vi "FM_WS_tool.vi"() -> ()   [LabVIEW 2013]
uses:
  <vilib>/NI VeriStand/Execution/Workspace/NI_VS Workspace ExecutionAPI.lvlib
  <vilib>/NI Veristand/Templates/Workspace Tool Support/Workspace Tool Response (String).ctl
  <vilib>/NI VeriStand/Templates/Workspace Tool Support/NI VeriStand - Workspace Tool Support.lvlib
  <vilib>/NI Veristand/Execution/Project/NI_VS Project ExecutionAPI.lvlib
  <vilib>/NI/AMC/AMC.lvlib
  <vilib>/NI Veristand/Execution/Project/Project Ref.ctl
  <vilib>/NI Veristand/Execution/Workspace/NI VeriStand - Get Multiple Channel Values.vi
  <vilib>/NI Veristand/Execution/Project/NI VeriStand - Send Workspace Tool Message (String).vi
  NationalInstruments.VeriStand.ClientAPI
  <vilib>/NI Veristand/Execution/Workspace/WorkspaceAPI.ctl
  NationalInstruments.VeriStand.SystemStorage
  _support/CustomTool_Data.ctl
  <vilib>/NI Veristand/Templates/Workspace Tool Support/Workspace Tool Response (Byte Array).ctl
  <vilib>/NI Veristand/Templates/Workspace Tool Support/Workspace Tool Message (Byte Array).ctl
  <vilib>/NI Veristand/Templates/Workspace Tool Support/Workspace Tool Message (String).ctl
  <vilib>/NI Veristand/Templates/Workspace Tool Support/Workspace Tool Message Bus.ctl
panel:
  out "value sent":dbl
  out "Execution:State (Before)":T1(ring)
  in  "Send Message To Service":bool
  in  "Launch Service":bool
  out "Send Error":errorcluster
  out "SaveSystemStorageFile":bool
  in  "Destination":path
  in  "Save As":bool
  in  "NIVS.Project Doc":refnum<k24>
  in  "Data":string
  out "Command":string
  out "Data":string
  in  "Command":string="Shut Down"
  in  "Custom Tool Path":string="..\\Workspace.vi"
  in  "Send":bool
  out "ShutDown Command?":bool
  in  "NIVS.Message Bus":T2
  in  "NIVS.ProjectRoot":refnum<k24>
  out "Commands Received":i32
  in  "Stop":bool
  in  "NIVS.System Definition Root":refnum<k24>
  in  "NIVS.Project File Path":path
  in  "NIVS.Workspace Event":refnum<event-registration>
  out "System Times":dbl[](array[numeric]) format="%<%H:%M:%S%3u>t"
  in  "NIVS.Gateway IP Address":string
  in  "NIVS.INI File Path":path
  # "Incoming Commands"
  # "Outgoing Commands"
  # "Status"
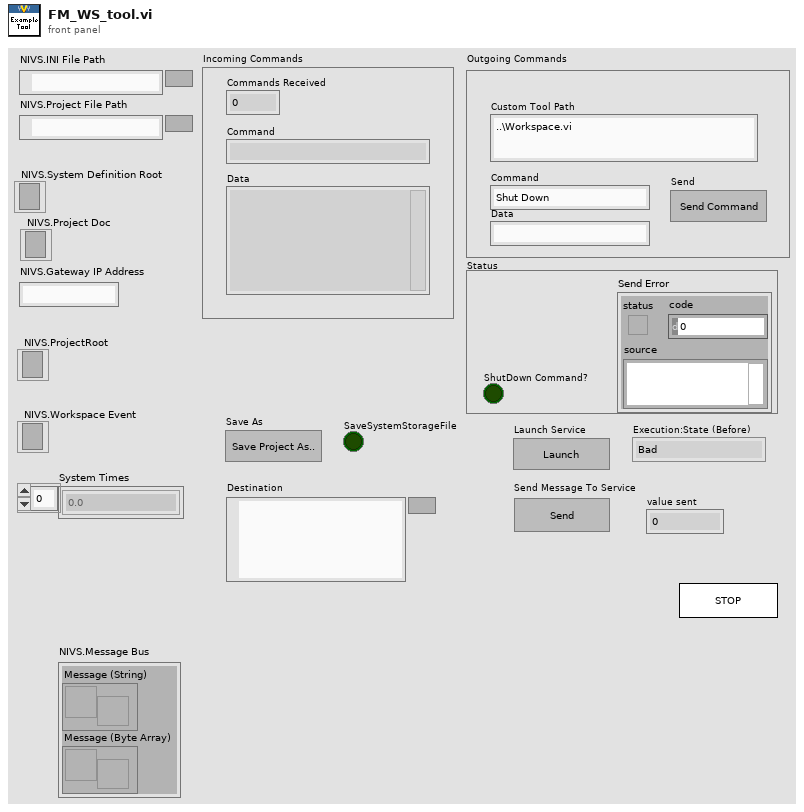
[diagram p1: front panel]
types:
  T1 = enum32{"Bad", "Idle", "Run top level", "Running"}
  T2 = typedef "NI VeriStand - Workspace Tool Support.lvlib/Workspace Tool Message Bus.ctl" = cluster{"Message (String)":refnum<user-event>, "Message (Byte Array)":refnum<user-event>}
  T3 = typedef "CustomTool_Data.ctl" = cluster{"Project Ref":T4, "Log File":path, "WorkspaceManager  out":T5, "NIVS.Project File Path":path, "NIVS.Project Doc":refnum<k24>, "Service Ref":refnum<vi>, "Service Name":string}
  T4 = typedef "NI_VS Project ExecutionAPI.lvlib/Project Ref.ctl" = refnum<k24>
  T5 = typedef "NI_VS Workspace ExecutionAPI.lvlib/WorkspaceAPI.ctl" = refnum<k24>
  T6 = typedef "NI_VS Workspace ExecutionAPI.lvlib/SystemStateEventRef.ctl" = cluster{"CustDatRef":refnum<user-event>, "EvtRef":refnum<k27>}
  T7 = typedef "NI_VS Workspace ExecutionAPI.lvlib/SystemStateRegEventRef.ctl" = refnum<event-registration>
  T8 = typedef "AMC.lvlib/Message Queue.ctl" = refnum<queue>
  T9 = cluster{"NIVS.Workspace Event":refnum<event-registration>, "SystemChangeEventRef":T7, "Event Registration Refnum":refnum<event-registration>}
  T10 = typedef "NI VeriStand - Workspace Tool Support.lvlib/Workspace Tool Response (String).ctl" = cluster{"Response":string, "Error":errorcluster}
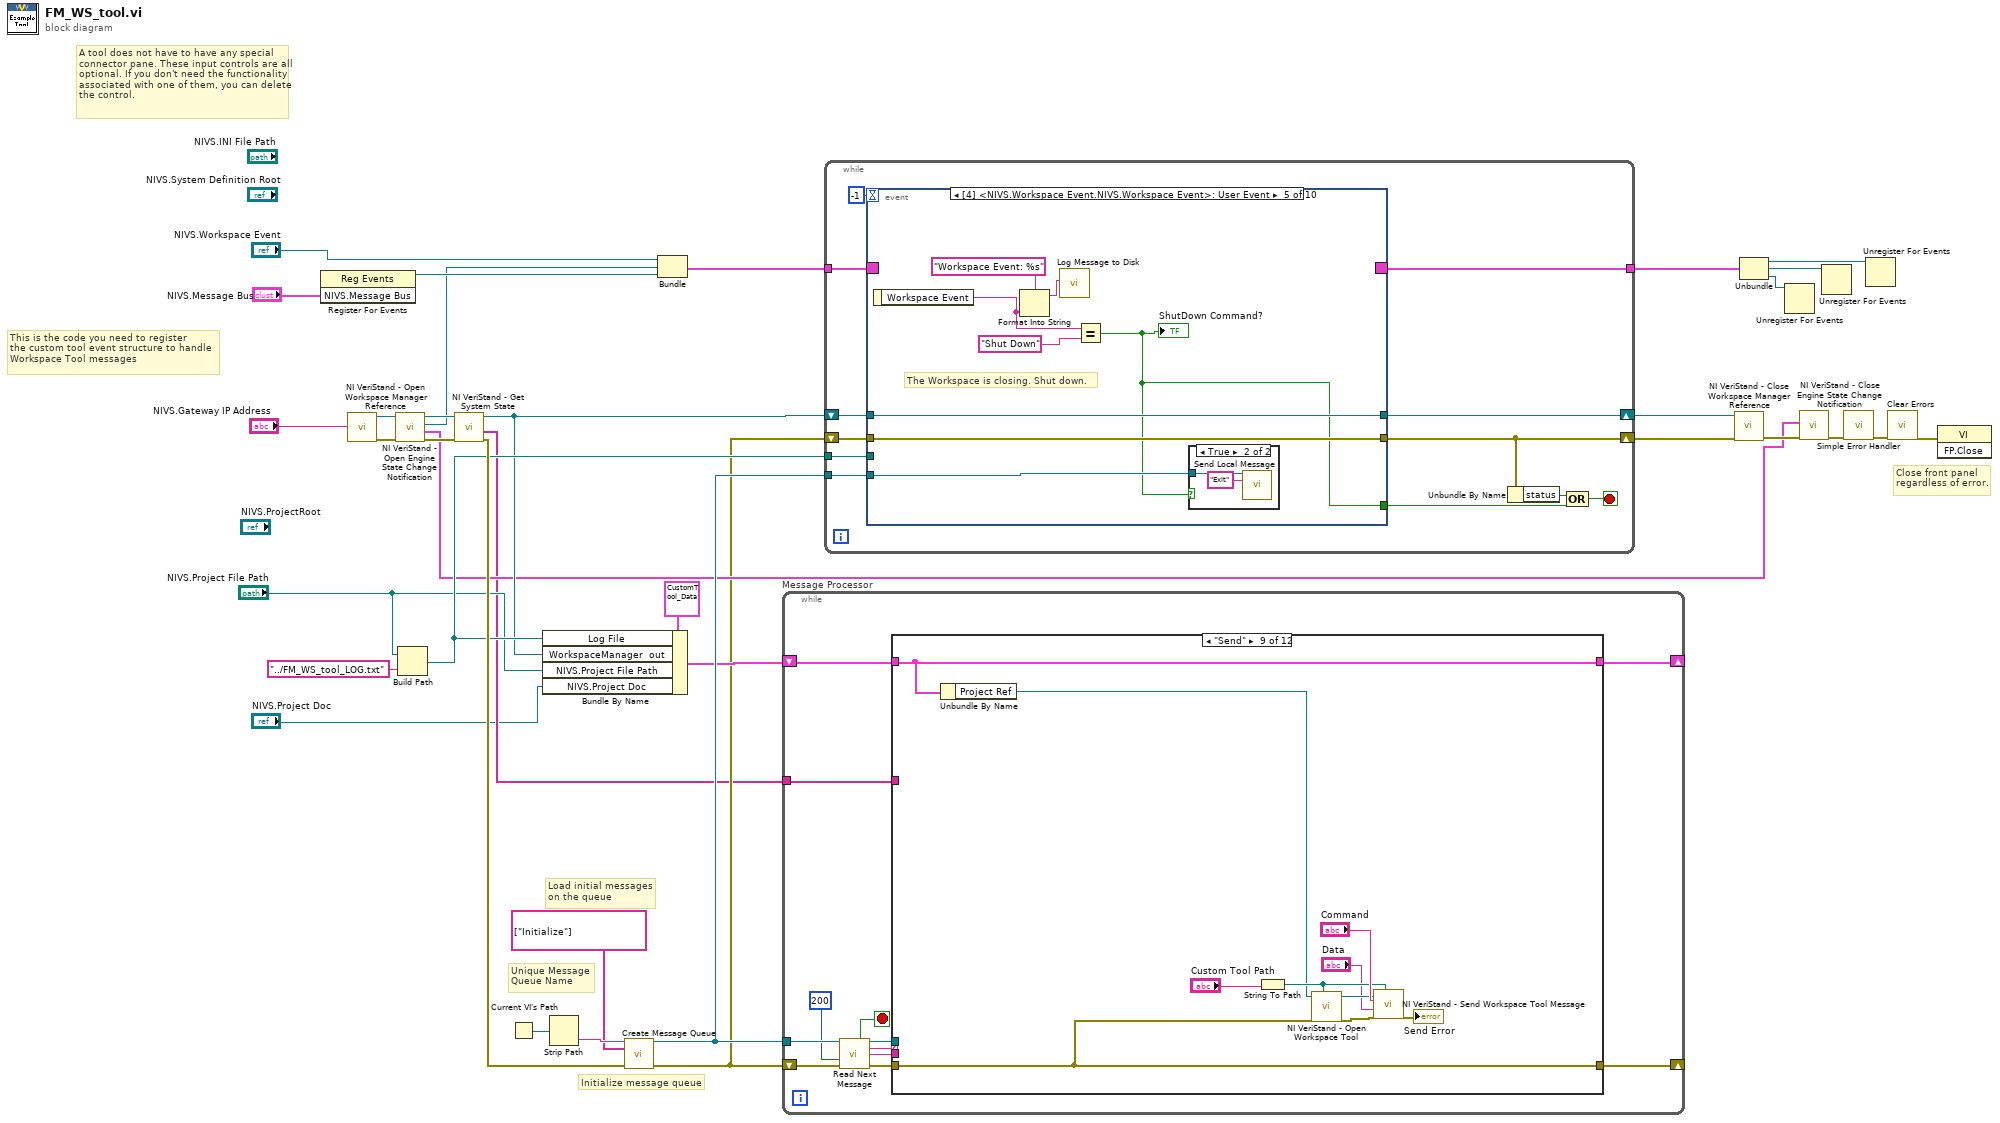
[diagram p0: block diagram]
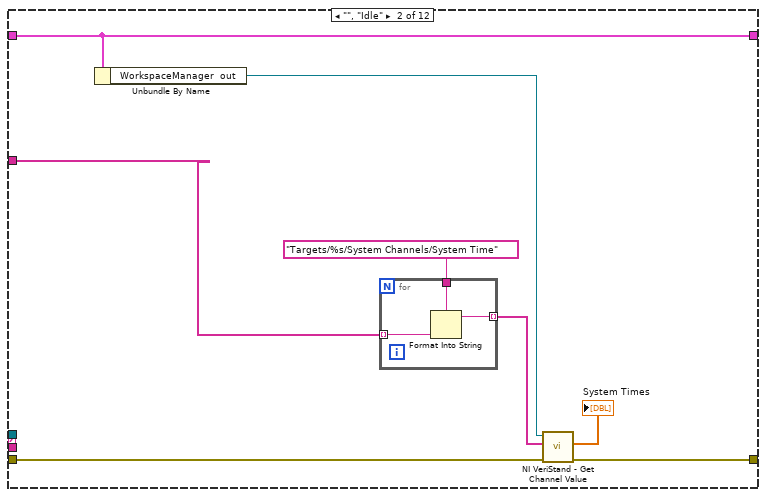
[diagram p3: hidden frame]
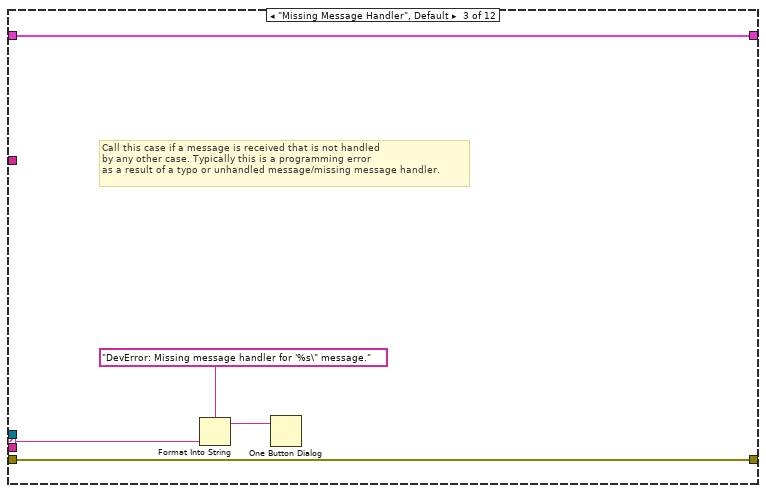
[diagram p4: hidden frame]
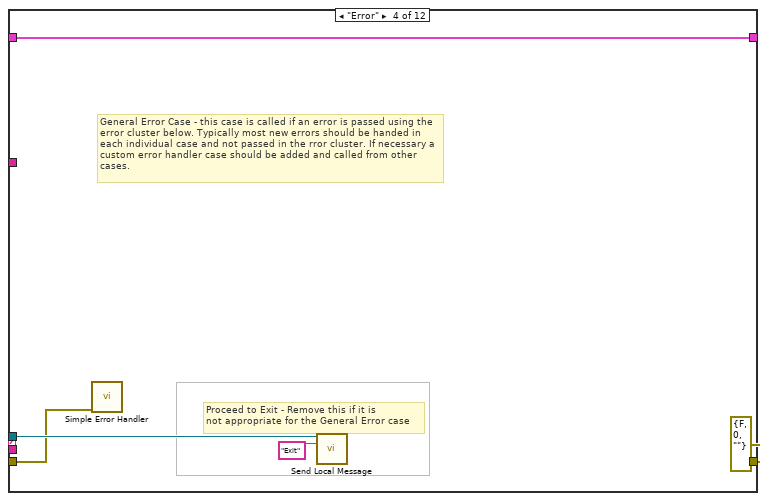
[diagram p5: hidden frame]
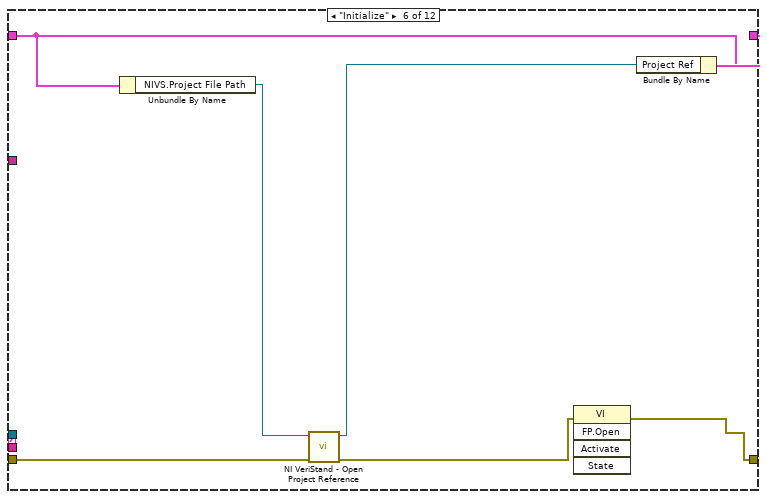
[diagram p7: hidden frame]
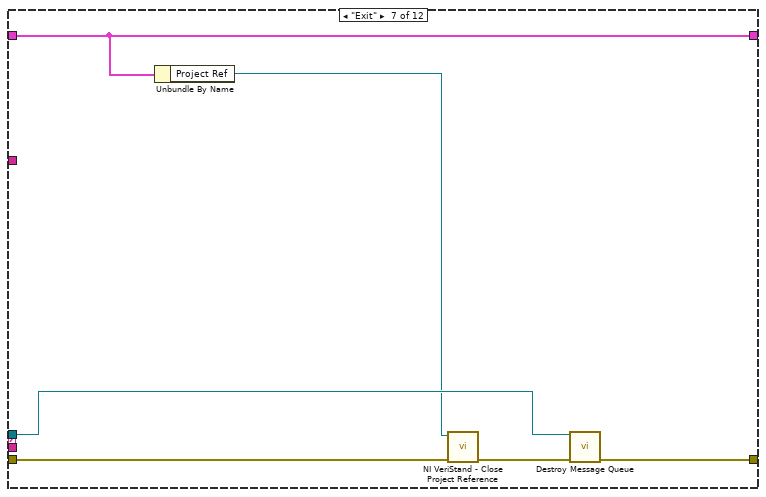
[diagram p8: hidden frame]
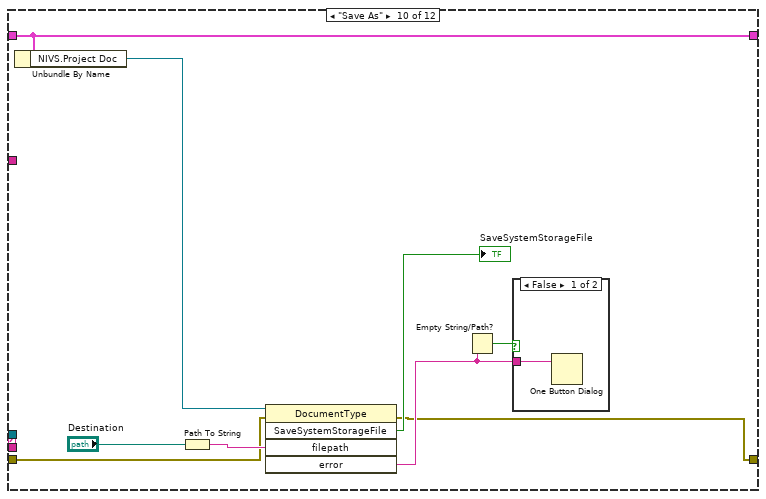
[diagram p10: hidden frame]
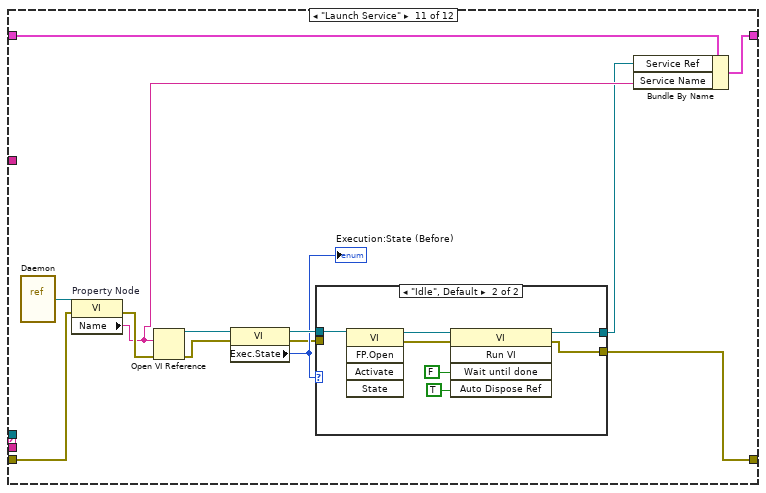
[diagram p12: hidden frame]
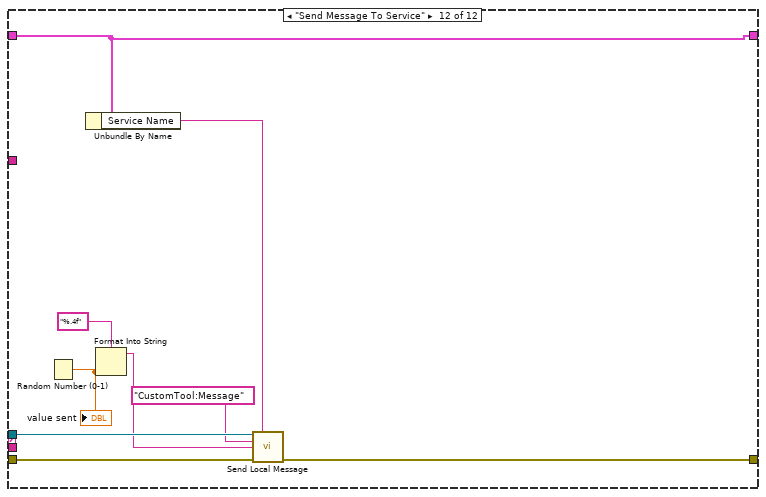
[diagram p14: hidden frame]
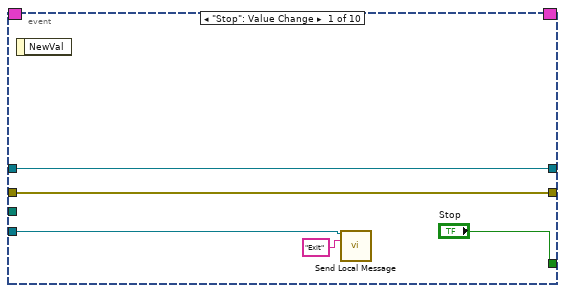
[diagram p15: hidden frame]
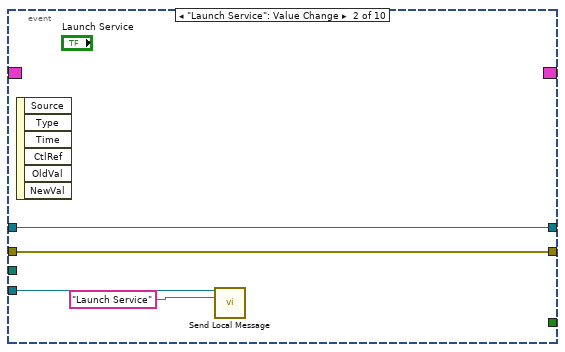
[diagram p16: hidden frame]
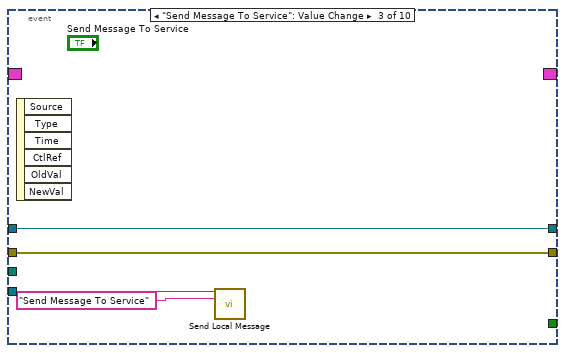
[diagram p17: hidden frame]
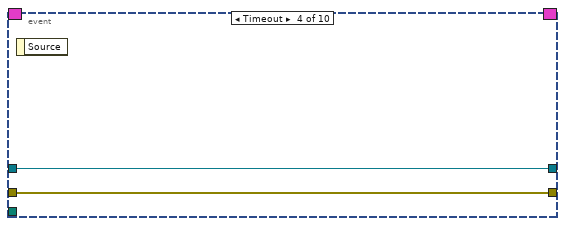
[diagram p18: hidden frame]
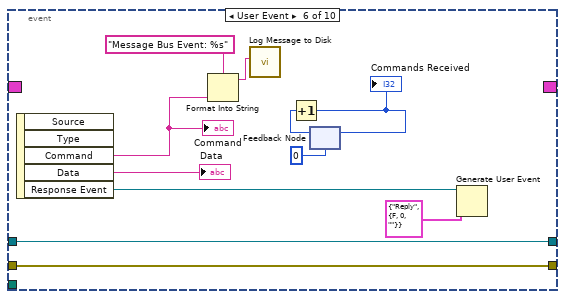
[diagram p20: hidden frame]
diagram:
  # "Initialize message queue"
  # "Unique Message\nQueue Name"
  # "Load initial messages\non the queue"
  # "This is the code you need to register \nthe custom tool event structure to handle\nWorkspace Tool messages"
  # "A tool does not have to have any special connector pane. These input controls are all optional. If you don't need the functionality associated with one of them, you can delete the control."
  # "Close front panel\nregardless of error."
  n1 = register-events("NIVS.Message Bus") -> (reference out=w24:refnum<event-registration>)  [unwired: 2 in, 1 out]
  n2 = call <vilib>:"NI VeriStand - Open Workspace Manager Reference.vi"("Gateway IP Address (\"\": localhost)"="NIVS.Gateway IP Address") -> ("error out"=w15:errorcluster, "WorkspaceManager"=w16:T5)  [unwired: 9 in]
  n3 = call <vilib>:"NI VeriStand - Open Engine State Change Notification.vi"("error in (no error)"=w15, "WorkspaceManager in"=w16) -> ("error out"=w17:errorcluster, "SystemStateRefs"=w5:T6, "SystemChangeEventRef"=w14:T7, "WorkspaceManager out"=w18:T5)  [unwired: 6 in]
  n4 = Build Path(base path="NIVS.Project File Path", name or relative path="../FM_WS_tool_LOG.txt") -> (appended path=w7:path)
  n5 = call <vilib>:"NI VeriStand - Get System State.vi"("error in (no error)"=w17, "WorkspaceManager in"=w18) -> ("error out"=w13:errorcluster, "Targets"=w2:string[], "WorkspaceManager  out"=w6:T5)  [unwired: 5 in, 2 out]
  n6 = Current VI's Path() -> (path=w22:path)
  n7 = Bundle By Name(cluster=T3 {"Project Ref"=refnum, "Log File"=path "", "WorkspaceManager  out"=refnum, "NIVS.Project File Path"=path "", "NIVS.Project Doc"=refnum, "Service Ref"=refnum, "Service Name"=""}, "Log File"=w7, "WorkspaceManager  out"=w6, "NIVS.Project File Path"="NIVS.Project File Path", "NIVS.Project Doc"="NIVS.Project Doc") -> (w8:T3)
  n8 = Strip Path(path=w22) -> (name=w21:string)  [unwired: 1 out]
  n9 = call <vilib>:"Create Message Queue.vi"("message queue name"=w21, "initial message names"=string[] ["Initialize"], "error in"=w13) -> ("message queue out"=w11:T8, "error out"=w4:errorcluster)  [unwired: 11 in]
  n10 = Bundle("NIVS.Workspace Event"="NIVS.Workspace Event", "SystemChangeEventRef"=w14, "Event Registration Refnum"=w24) -> (w33:T9)  [unwired: 1 in]
  n11 = while "Message Processor" {
    shift-left: w4 -> [w41]
    shift-right: [w45] -> _
    tunnel: w11 -> [w42]
    shift-left: w8 -> [w47]
    shift-right: [w46] -> _
    tunnel: w2 -> [w36]
    stop <- w44 stop-if-true
    n12 = call <vilib>:"Read Next Message.vi"("message queue in"=w42, "timeout (1 ms)"=200, "error in"=w41) -> ("exit process?"=w44:bool, "message queue out"=w43:T8, "message name"=w39:string, "message value"=w38:string, "error out"=w40:errorcluster)  [unwired: 5 in, 3 out]
    n13 = case shown="\"Send\"" w39 {
      selector: w39 -> [_ _ w63 _ _ _ _ _ _ _ _ _]
      tunnel: [w49 w57 w65 w70 w72 w78 w83 w87 w89 w99 w108 w131] -> w46
      tunnel: w47 -> [w49 w57 w65 w70 w72 w77 w83 w87 w89 w99 w111 w131]
      tunnel: w43 -> [_ _ _ w68 _ _ w85 _ _ _ _ w138]
      tunnel: w40 -> [w48 w54 w64 w66 w71 w79 w82 w86 w91 w101 w114 w135]
      tunnel: [w48 w53 w64 errorcluster {"status"=FALSE, "code"=0, "source"=""} ("error out") w71 w73 w84 w86 w91 w100 w112 w130] -> w45
      tunnel: w38 -> [_ _ _ _ _ _ _ _ _ _ _ _]
      tunnel: w36 -> [_ w50 _ _ _ _ _ _ _ _ _ _]
      frame "---------- Framework Operations ----------" {
        # "Dummy case to add a seperator in the Case Structure menu"
      }
      frame "", "Idle" {
        n14 = Unbundle By Name(w57) -> ("WorkspaceManager  out"=w51:T5)
        n15 = for {
          tunnel: "Targets/%s/System Channels/System Time" ("format string") -> [w60]
          tunnel: [w59] -> w56 mode=indexing
          tunnel: w50 -> [w58] mode=indexing
          n16 = Format Into String(format string=w60, w58) -> (resulting string=w59:string)  [unwired: 2 in, 1 out]
        }
        n17 = call-poly <vilib>:"NI VeriStand - Get Channel Value.vi"("error in (no error)"=w54, "Channels"=w56, "WorkspaceManager in"=w51) -> ("error out"=w53:errorcluster, "Values"=→"System Times":dbl[])  [unwired: 6 in, 1 out]
      }
      frame "Missing Message Handler", Default {
        # "Call this case if a message is received that is not handled \nby any other case. Typically this is a programming error\nas a result of a typo or unhandled message/missing message handler."
        n18 = Format Into String(format string="DevError: Missing message handler for '%s\" message." ("message"), w63) -> (resulting string=w61:string)  [unwired: 2 in, 1 out]
        n19 = One Button Dialog(message=w61) -> ()  [unwired: 2 out]
      }
      frame "Error" {
        # "Proceed to Exit - Remove this if it is\nnot appropriate for the General Error case"
        # "General Error Case - this case is called if an error is passed using the error cluster below. Typically most new errors should be handed in each individual case and not passed in the rror cluster. If necessary a custom error handler case should be added and called from other cases."
        n20 = call <vilib>:"Simple Error Handler.vi"("error in (no error)"=w66) -> ()  [unwired: 1 in, 8 out]
        n21 = call <vilib>:"Send Local Message.vi"("message queue in"=w68, "message name"="Exit") -> ()  [unwired: 11 in, 3 out]
      }
      frame "---------- Generic Operations ----------" {
        # "Dummy case to add a seperator in the Case Structure menu"
      }
      frame "Initialize" {
        n22 = Unbundle By Name(w77) -> ("NIVS.Project File Path"=w76:path)
        n23 = call <vilib>:"NI VeriStand - Open Project Reference.vi"("error in (no error)"=w79, "Project File Path"=w76) -> ("error out"=w74:errorcluster, "Project Ref"=w75:T4)  [unwired: 8 in]
        n24 = invoke class="VI" method="FP.Open"(error in=w74) -> (error out=w73:errorcluster)  [unwired: 4 in, 4 out]
        n25 = Bundle By Name(cluster=w77, "Project Ref"=w75) -> (w78:T3)
      }
      frame "Exit" {
        n26 = Unbundle By Name(w83) -> ("Project Ref"=w80:T4)
        n27 = call <vilib>:"NI VeriStand - Close Project Reference.vi"("error in (no error)"=w82, "Project Ref"=w80) -> ("error out"=w81:errorcluster)  [unwired: 9 in]
        n28 = call <vilib>:"Destroy Message Queue.vi"("message queue in"=w85, "error in"=w81) -> ("error out"=w84:errorcluster)  [unwired: 11 in, 2 out]
      }
      frame "---------- Application Operations ----------" {
        # "Dummy case to add a seperator in the Case Structure menu"
      }
      frame "Send" {
        n29 = Unbundle By Name(w89) -> ("Project Ref"=w88:T4)
        n30 = String To Path(string="Custom Tool Path") -> (path=w93:path)
        n31 = call <vilib>:"NI VeriStand - Open Workspace Tool.vi"("Workspace Tool Path"=w93, "error in (no error)"=w91, "Project Ref in"=w88) -> ("error out"=w94:errorcluster, "Project Ref out"=w95:T4)  [unwired: 7 in]
        n32 = call-poly <vilib>:"NI VeriStand - Send Workspace Tool Message.vi"("Workspace Tool Path"=w93, "error in (no error)"=w94, "Data"="Data", "Command"="Command", "Project Ref in"=w95) -> ("error out"=→"Send Error":errorcluster)  [unwired: 4 in, 2 out]
      }
      frame "Save As" {
        n33 = Unbundle By Name(w99) -> ("NIVS.Project Doc"=w98:refnum<k24>)
        n34 = Path To String(path="Destination") -> (string=w102:string)
        n35 = invoke class="DocumentType" method="SaveSystemStorageFile"(reference=w98, error in=w101, "filepath"=w102) -> (error out=w100:errorcluster, "SaveSystemStorageFile"=→"SaveSystemStorageFile":bool, "error"=w103:string)  [unwired: 2 in, 2 out]
        n36 = Empty String/Path?(string/path=w103) -> (empty?=w104:bool)
        n37 = case shown="False" w104 {
          tunnel: w103 -> [w107 _]
          frame False {
            n38 = One Button Dialog(message=w107) -> ()  [unwired: 1 in, 1 out]
          }
          frame True {
          }
        }
      }
      frame "Launch Service" {
        n39 = vi-ref "Daemon.vi"() -> (w120:refnum<vi>)
        n40 = property on="Property Node" class="VI"(reference=w120, error in=w114) -> (error out=w113:errorcluster, "Name"=w110:string)  [unwired: 1 out]
        n41 = Open VI Reference(vi path=w110, error in (no error)=w113) -> (vi reference=w119:refnum<vi>, error out=w118:errorcluster)  [unwired: 4 in]
        n42 = property class="VI"(reference=w119, error in=w118) -> (reference out=w117:refnum<vi>, error out=w115:errorcluster, "Exec.State"=w116:T1)
        "Execution:State (Before)" <- w116
        n43 = case shown="\"Idle\", Default" w116 {
          tunnel: w117 -> [w122 w125]
          tunnel: [w122 w124] -> w109
          tunnel: w115 -> [w121 _]
          tunnel: [w121 w123] -> w112
          frame "Run top level" {
          }
          frame "Idle", Default {
            n44 = invoke class="VI" method="FP.Open"(reference=w125) -> (reference out=w127:refnum<vi>, error out=w126:errorcluster)  [unwired: 4 in, 3 out]
            n45 = invoke class="VI" method="Run VI"(reference=w127, error in=w126, "Wait until done"=FALSE ("Auto Dispose Reference"), "Auto Dispose Ref"=TRUE ("Auto Dispose Reference")) -> (reference out=w124:refnum<vi>, error out=w123:errorcluster)  [unwired: 1 in, 3 out]
          }
        }
        n46 = Bundle By Name(cluster=w111, "Service Ref"=w109, "Service Name"=w110) -> (w108:T3)
      }
      frame "Send Message To Service" {
        n47 = Random Number (0-1)() -> (number: 0 to 1=w134:dbl)
        "value sent" <- w134
        n48 = Unbundle By Name(w131) -> ("Service Name"=w137:string)
        n49 = Format Into String(format string="%.4f", w134) -> (resulting string=w132:string)  [unwired: 2 in, 1 out]
        n50 = call <vilib>:"Send Local Message.vi"("message queue in"=w138, "receiver process (\"\" - local)"=w137, "message name"="CustomTool:Message", "message value"=w132, "error in"=w135) -> ("error out"=w130:errorcluster)  [unwired: 8 in, 2 out]
      }
    }
  }
  n51 = while {
    tunnel: w33 -> [w150]
    tunnel: [w149] -> w32
    shift-right: [w144] -> w34
    shift-left: w4 -> [w147]
    shift-right: [w146] -> w35
    shift-left: w6 -> [w148]
    tunnel: w11 -> [w140]
    tunnel: w7 -> [w139]
    stop <- w142 stop-if-true
    n52 = event shown="[4] <NIVS.Workspace Event.NIVS.Workspace Event>: User Event" {
      selector: w150 -> [_ _ _ _ _ _ _ _ _ _]
      dyn-events: [_ _ _ _ _ _ _ _ _ _] -> w149
      timeout: -1 -> [_ _ _ _ _ _ _ _ _ _]
      tunnel: ["Stop" _ _ _ w166 _ w187 w193 _ _] -> w143
      tunnel: w148 -> [w154 w158 w162 w165 w172 w185 w190 w196 w202 w206]
      tunnel: w147 -> [w155 w159 w163 w164 w173 w186 w191 w197 w203 w207]
      tunnel: [w155 w159 w163 w164 w173 w186 w191 w197 w203 w207] -> w144
      tunnel: [w154 w158 w162 w165 w172 w185 w190 w196 w202 w206] -> w146
      tunnel: w140 -> [w151 w157 w161 _ w167 _ w189 w192 w201 w205]
      tunnel: w139 -> [_ _ _ _ _ _ _ _ _ _]
      event "Stop": Value Change {
        n53 = event-data() -> ()  [unwired: 1 in, 1 out]
        n54 = call <vilib>:"Send Local Message.vi"("message queue in"=w151, "message name"="Exit") -> ()  [unwired: 11 in, 3 out]
      }
      event "Launch Service": Value Change {
        n55 = event-data() -> ()  [unwired: 1 in, 6 out]
        n56 = call <vilib>:"Send Local Message.vi"("message queue in"=w157, "message name"="Launch Service") -> ()  [unwired: 11 in, 3 out]
      }
      event "Send Message To Service": Value Change {
        n57 = event-data() -> ()  [unwired: 1 in, 6 out]
        n58 = call <vilib>:"Send Local Message.vi"("message queue in"=w161, "message name"="Send Message To Service") -> ()  [unwired: 11 in, 3 out]
      }
      event Timeout {
        n59 = event-data() -> ()  [unwired: 1 in, 1 out]
      }
      event User Event {
        # "The Workspace is closing. Shut down."
        n60 = event-data() -> ("Workspace Event"=w169:string)  [unwired: 1 in]
        n61 = Format Into String(format string="Workspace Event: %s", w169) -> (resulting string=w168:string)  [unwired: 2 in, 1 out]
        n62 = call "Log Message to Disk.vi"("Message"=w168) -> ()  [unwired: 10 in, 1 out]
        n63 = Equal?(x=w169, y="Shut Down") -> (x = y?=w166:bool)
        "ShutDown Command?" <- w166
        n64 = case shown="True" w166 {
          tunnel: w167 -> [_ w175]
          frame False {
          }
          frame True {
            n65 = call <vilib>:"Send Local Message.vi"("message queue in"=w175, "message name"="Exit") -> ()  [unwired: 11 in, 3 out]
          }
        }
      }
      event User Event {
        n66 = event-data() -> ("Command"=w182:string, "Data"=→"Data":string, "Response Event"=w178:refnum<user-event>)  [unwired: 1 in, 2 out]
        "Command" <- w182
        n67 = Format Into String(format string="Message Bus Event: %s", w182) -> (resulting string=w183:string)  [unwired: 2 in, 1 out]
        n68 = call "Log Message to Disk.vi"("Message"=w183) -> ()  [unwired: 10 in, 1 out]
        n69 = feedback #1(0) -> (w181:i32)
        n70 = Increment(x=w181) -> (x+1=w180:i32)
        "Commands Received" <- w180
        n71 = feedback-in #1(w180) -> ()
        n72 = Generate User Event(user event=w178, event data cluster=T10 {"Response"="Reply", "Error"={"status"=FALSE, "code"=0, "source"=""}} ("event data")) -> ()  [unwired: 2 in, 2 out]
      }
      event Panel Close? {
        w187 = TRUE ("Discard?")
        n73 = event-data() -> ()  [unwired: 1 in, 1 out]
        n74 = call <vilib>:"Send Local Message.vi"("message queue in"=w189, "message name"="Exit") -> ()  [unwired: 11 in, 3 out]
        n75 = event-data("Discard?"=w187) -> ()  [unwired: 1 in, 1 out]
      }
      event User Event {
        # "The VeriStand Gateway is disconnecting from the targets. Shut down."
        n76 = event-data() -> ("SystemStateChange"=w195:string)  [unwired: 1 in]
        n77 = Equal?(x=w195, y="Stop Configuration") -> (x = y?=w193:bool)
        n78 = case shown="True" w193 {
          tunnel: w192 -> [_ w199]
          frame False {
          }
          frame True {
            n79 = call <vilib>:"Send Local Message.vi"("message queue in"=w199, "message name"="Exit") -> ()  [unwired: 11 in, 3 out]
          }
        }
      }
      event "Send": Value Change {
        n80 = event-data() -> ()  [unwired: 1 in, 1 out]
        n81 = call <vilib>:"Send Local Message.vi"("message queue in"=w201, "message name"="Send") -> ()  [unwired: 11 in, 3 out]
      }
      event "Save As": Value Change {
        # ".nivsscren\n.nivssysdef"
        n82 = event-data() -> ()  [unwired: 1 in, 2 out]
        n83 = call <vilib>:"Send Local Message.vi"("message queue in"=w205, "message name"="Save As") -> ()  [unwired: 11 in, 3 out]
      }
    }
    n84 = Unbundle By Name(w144) -> ("status"=w145:bool)
    n85 = Compound Arithmetic op=OR(w145, w143) -> (w142:bool)
  }
  n86 = call <vilib>:"NI VeriStand - Close Workspace Manager Reference.vi"("error in (no error)"=w34, "WorkspaceManager"=w35) -> ("error out"=w29:errorcluster)  [unwired: 9 in]
  n87 = Unbundle(w32) -> ("NIVS.Workspace Event"=w30:refnum<event-registration>, "SystemChangeEventRef"=w31:T7, "Event Registration Refnum"=w23:refnum<event-registration>)
  n88 = Unregister For Events(event registration refnum=w23) -> ()  [unwired: 1 in, 1 out]
  n89 = call <vilib>:"NI VeriStand - Close Engine State Change Notification.vi"("error in (no error)"=w29, "SystemStateRefs"=w5) -> ("error out"=w27:errorcluster)  [unwired: 9 in]
  n90 = Unregister For Events(event registration refnum=w31) -> ()  [unwired: 1 in, 1 out]
  n91 = call <vilib>:"Simple Error Handler.vi"("error in (no error)"=w27) -> ("error out"=w26:errorcluster)  [unwired: 4 in, 4 out]
  n92 = Unregister For Events(event registration refnum=w30) -> ()  [unwired: 1 in, 1 out]
  n93 = call <vilib>:"Clear Errors.vi"("error in (no error)"=w26) -> ("error out"=w25:errorcluster)  [unwired: 6 in]
  n94 = invoke class="VI" method="FP.Close"(error in=w25) -> ()  [unwired: 2 in, 3 out]
